vi "Write Network Protocol.vi"(8 "error in (no error)":errorcluster, 10 "Network Protocol":refnum<class "Network Protocol.lvclass">, 11 "Modbus API in":refnum<class "Modbus API.lvclass">) -> (0 "error out":errorcluster, 3 "Modbus API out":refnum<class "Modbus API.lvclass">)   [LabVIEW 2021, in "Modbus API.lvclass"]
uses:
  Modbus API.lvclass
  Network Protocol/Network Protocol.lvclass
  Modbus API.lvclass/Modbus API.ctl
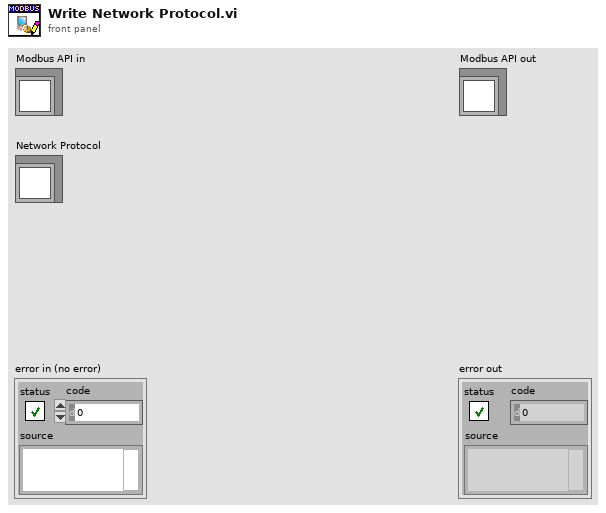
[diagram p1: front panel]
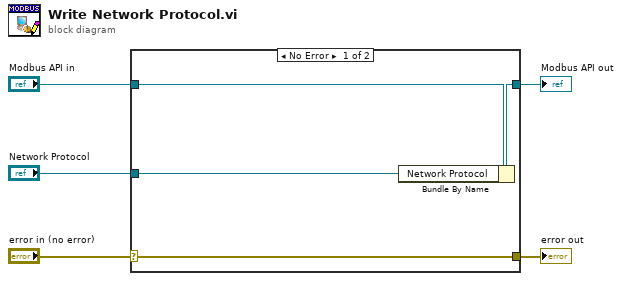
[diagram p0: block diagram]
diagram:
  n1 = case shown="No Error" "error in (no error)" {
    selector: "error in (no error)" -> [w9 w10]
    tunnel: [w9 w10] -> w4
    tunnel: [w7 w11] -> w2
    tunnel: "Modbus API in" -> [w8 w11]
    tunnel: "Network Protocol" -> [w6 _]
    frame No Error {
      n2 = Bundle By Name(cluster=w8, "Network Protocol"=w6) -> (w7:refnum<class "Modbus API.lvclass">)
    }
    frame Error {
    }
  }
  "error out" <- w4
  "Modbus API out" <- w2
